vi "Get Tunnel Direction.vi"(11 "Tunnel in":refnum<vi>) -> (3 "Tunnel Direction":enum16{"In-Going", "Out-Going"}(ring))   [LabVIEW 2023]
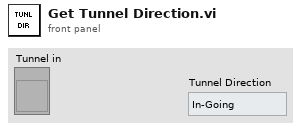
[diagram p1: front panel]
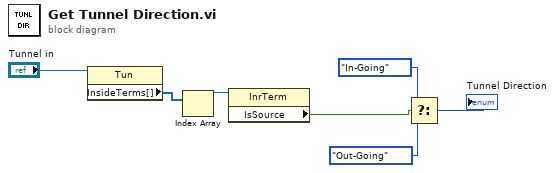
[diagram p0: block diagram]
diagram:
  n1 = property class="Tun"(reference="Tunnel in") -> ("InsideTerms[]"=w6:refnum<vi>[])  [unwired: 1 in, 2 out]
  n2 = Index Array(array=w6) -> (element=w7:refnum<vi>)  [unwired: 1 in]
  n3 = property class="InrTerm"(reference=w7) -> ("IsSource"=w4:bool)  [unwired: 1 in, 2 out]
  n4 = Select(t=enum16{"In-Going", "Out-Going"}."In-Going" ("Tunnel Direction"), s=w4, f=enum16{"In-Going", "Out-Going"}."Out-Going" ("Tunnel Direction")) -> (s? t:f=→"Tunnel Direction":enum16{"In-Going", "Out-Going"})
